vi "Depth section.vi"(11 "深度資訊(mm)":u16) -> (3 "Output section":u16)   [LabVIEW 2019, in "SR_2000.lvlib"]
uses:
  SR_2000.lvlib
panel:
  out "floor(x/y)":u16
  out "x-y*floor(x/y)":u16
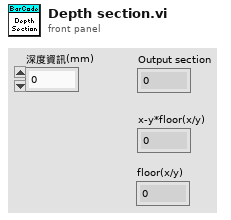
[diagram p1: front panel]
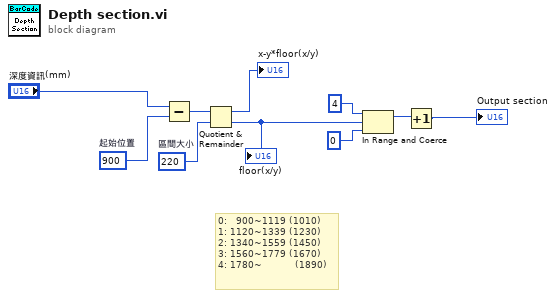
[diagram p0: block diagram]
diagram:
  w6 = u16 220  # 區間大小
  w4 = u16 900  # 起始位置
  # "0:   900~1119 (1010)\n1: 1120~1339 (1230)\n2: 1340~1559 (1450)\n3: 1560~1779 (1670)\n4: 1780~           (1890)"
  n1 = Subtract(x="深度資訊(mm)", y=w4) -> (x-y=w5:u16)
  n2 = Quotient & Remainder(x=w5, y=w6) -> (x-y*floor(x/y)=→"x-y*floor(x/y)":u16, floor(x/y)=w8:u16)
  "floor(x/y)" <- w8
  n3 = In Range and Coerce(upper limit=u16 4, x=w8, lower limit=u16 0) -> (coerced(x)=w3:u16)  [unwired: 1 out]
  n4 = Increment(x=w3) -> (x+1=→"Output section":u16)
